vi "Mixer.Open.vi"() -> (0 "success":bool)   [LabVIEW 2020]
uses:
  <vilib>/Utility/sysdir.llb/System Directory Type.ctl
  <vilib>/Utility/config.llb/Read Key (I32).vi
  <vilib>/Utility/config.llb/NI_LVConfig.lvlib
panel:
  out "error out":errorcluster
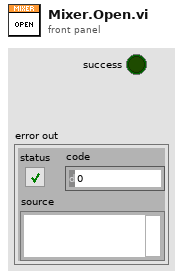
[diagram p1: front panel]
types:
  T1 = enum32{"Bad", "Idle", "Run top level", "Running"}
  T2 = enum32{"Invalid", "Standard", "Closed", "Hidden", "Minimized", "Maximized"}
  T3 = typedef "System Directory Type.ctl" = i32
  T4 = typedef "NI_LVConfig.lvlib/Config Data RefNum.ctl" = refnum<k1>
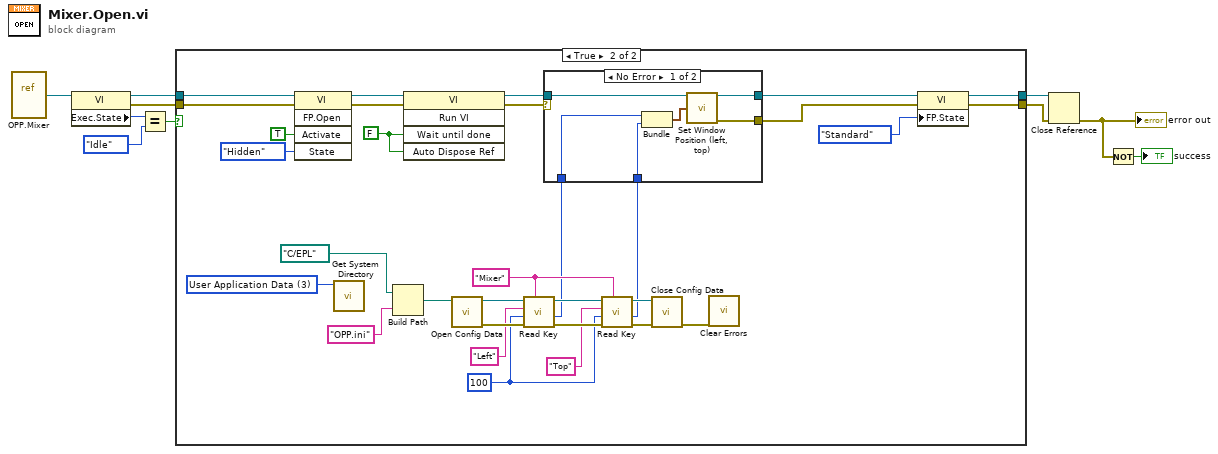
[diagram p0: block diagram]
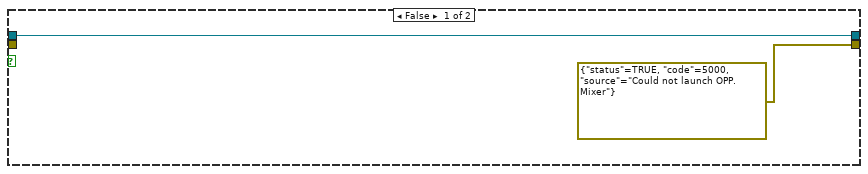
[diagram p2: hidden frame]
diagram:
  n1 = vi-ref "OPP.Mixer.vi"() -> (w5:refnum<vi>)
  n2 = property class="VI"(reference=w5) -> (reference out=w10:refnum<vi>, error out=w9:errorcluster, "Exec.State"=w4:T1)  [unwired: 1 in]
  n3 = Equal?(x=w4, y=T1."Idle" ("Execution:State")) -> (x = y?=w3:bool)
  n4 = case shown="True" w3 {
    tunnel: w10 -> [w12 w27]
    tunnel: w9 -> [_ w26]
    tunnel: [w12 w22] -> w8
    tunnel: [errorcluster {"status"=TRUE, "code"=5000, "source"="Could not launch OPP.Mixer"} ("error out") w21] -> w7
    frame False {
    }
    frame True {
      w25 = FALSE ("Wait Until Done")
      w29 = 100 ("default value")
      w34 = "Mixer" ("section")
      w30 = T3 3 items=["User Home"=0, "User Desktop"=1, "User Documents"=2, "User Application Data"=3, "User Preferences"=4, "User Temporary"=5, "Public Documents"=6, "Public Application Data"=7, "Public Preferences"=8, "Public Cache"=13, "System Core Libraries"=9, "System Installed Libraries"=10, "Application Files"=11, "Boot Volume Root"=12] ("system directory type")
      n5 = invoke class="VI" method="FP.Open"(reference=w27, error in=w26, "Activate"=TRUE ("Activate?"), "State"=T2."Hidden") -> (reference out=w24:refnum<vi>, error out=w23:errorcluster)  [unwired: 1 in, 3 out]
      n6 = call <vilib>:"Get System Directory.vi"("system directory type"=w30) -> ()  [unwired: 10 in, 1 out]
      n7 = Build Path(base path=path "C:/EPL", name or relative path="OPP.ini") -> (appended path=w41:path)
      n8 = invoke class="VI" method="Run VI"(reference=w24, error in=w23, "Wait until done"=w25, "Auto Dispose Ref"=w25) -> (reference out=w19:refnum<vi>, error out=w14:errorcluster)  [unwired: 1 in, 3 out]
      n9 = call <vilib>:"Open Config Data.vi"("configuration file path"=w41) -> ("error out"=w38:errorcluster, "refnum"=w40:T4)  [unwired: 8 in, 1 out]
      n10 = call-poly <vilib>:"Read Key.vi"("section"=w34, "error in (no error)"=w38, "default value"=w29, "key"="Left", "refnum"=w40) -> ("error out"=w37:errorcluster, "value"=w18:i32, "refnum out"=w39:T4)  [unwired: 3 in, 1 out]
      n11 = call-poly <vilib>:"Read Key.vi"("section"=w34, "error in (no error)"=w37, "default value"=w29, "key"="Top", "refnum"=w39) -> ("error out"=w36:errorcluster, "value"=w17:i32, "refnum out"=w35:T4)  [unwired: 3 in, 1 out]
      n12 = case shown="No Error" w14 {
        selector: w14 -> [_ w50]
        tunnel: w19 -> [w49 w51]
        tunnel: w18 -> [w48 _]
        tunnel: w17 -> [w47 _]
        tunnel: [w45 w51] -> w16
        tunnel: [w44 w50] -> w15
        frame No Error {
          n13 = Bundle("value"=w48, "value"=w47) -> (w46:cluster{"value":i32, "value":i32})  [unwired: 1 in]
          n14 = call "Set Window Position (left, top).vi"("VI in"=w49, "Coords"=w46) -> ("VI out"=w45:refnum<vi>, "error out"=w44:errorcluster)  [unwired: 12 in]
        }
        frame Error {
        }
      }
      n15 = call <vilib>:"Close Config Data.vi"("error in (no error)"=w36, "refnum"=w35) -> ("error out"=w28:errorcluster)  [unwired: 8 in, 1 out]
      n16 = call <vilib>:"Clear Errors.vi"("error in (no error)"=w28) -> ()  [unwired: 5 in, 2 out]
      n17 = property class="VI"(reference=w16, error in=w15, "FP.State"=T2."Standard" ("Front Panel Window:State")) -> (reference out=w22:refnum<vi>, error out=w21:errorcluster)
    }
  }
  n18 = Close Reference(reference=w8, error in (no error)=w7) -> (error out=w1:errorcluster)
  "error out" <- w1
  n19 = Not(x=w1) -> (.not. x?=→"success":bool)
